vi "Core-Init.vi"(10 "Class Return Notifier":refnum<notifier>, 11 "Engine in":refnum<class "Engine.lvclass">) -> (0 "error out":errorcluster, 3 "Engine out":refnum<class "Engine.lvclass">)   [LabVIEW 2024, in "GLF.lvlib" / "Engine.lvclass"]
uses:
  Engine.lvclass
  IAmGLF/IAmGLF.lvclass
  Window/Window.lvclass
  Engine.lvclass/Engine.ctl
  C:/Users/saukko/Dev/GLF/Sources/GLF/IAmEngine/IAmEngine.lvclass
  C:/Users/saukko/Dev/GLF/Sources/GLF/IAmGLF/IAmGLF.lvclass
  C:/Users/saukko/Dev/GLF/Sources/GLF/Engine/Engine.lvclass
  <vilib>/Saukko/LV SDL3/Sources/SDL3/Init/Init.lvlib
  Command--enum.ctl
  Command--cluster.ctl
  <vilib>/Saukko/LV SDL3/Sources/SDL3/Init/InitFlags--ring.ctl
  <vilib>/Saukko/LV SDL3/Sources/SDL3/Video/Video.lvlib
  DVR--cluster.ctl
  Metrics--cluster.ctl
  Context--cluster.ctl
  Config--cluster.ctl
  VSync--enum.ctl
  Command--queue.ctl
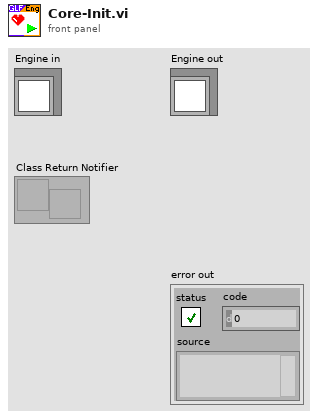
[diagram p1: front panel]
types:
  T1 = typedef "GLF.lvlib/Engine.lvclass/VSync--enum.ctl" = enum16{"Disabled", "Enabled", "Adaptative"}
  T2 = typedef "GLF.lvlib/Engine.lvclass/DVR--cluster.ctl" = cluster{"CMD Queue":T3, "Config":T4, "Ctxt":T5, "Metrics":T6, "GLF Instances":set{refnum<class "IAmGLF.lvclass">}, "Window Instances":map{i64, refnum<class "Window.lvclass">}}
  T3 = typedef "GLF.lvlib/Engine.lvclass/Command--queue.ctl" = refnum<queue>
  T4 = typedef "GLF.lvlib/Engine.lvclass/Config--cluster.ctl" = cluster{"Quit On Last Window Closed":bool, "VSync":T1, "FPS Target":dbl}
  T5 = typedef "GLF.lvlib/Engine.lvclass/Context--cluster.ctl" = cluster{"Ticks Begin":u64, "VSync Enabled":bool}
  T6 = typedef "GLF.lvlib/Engine.lvclass/Metrics--cluster.ctl" = cluster{"Uptime [ms]":u64, "Loop Time [ms]":u64}
  T7 = typedef "SDL3.lvlib/Init.lvlib/InitFlags--ring.ctl" = u32
  T8 = typedef "GLF.lvlib/Engine.lvclass/Command--cluster.ctl" = cluster{"Cmd":T9, "Data":variant}
  T9 = typedef "GLF.lvlib/Engine.lvclass/Command--enum.ctl" = enum16{"Quit", "Register Window"}
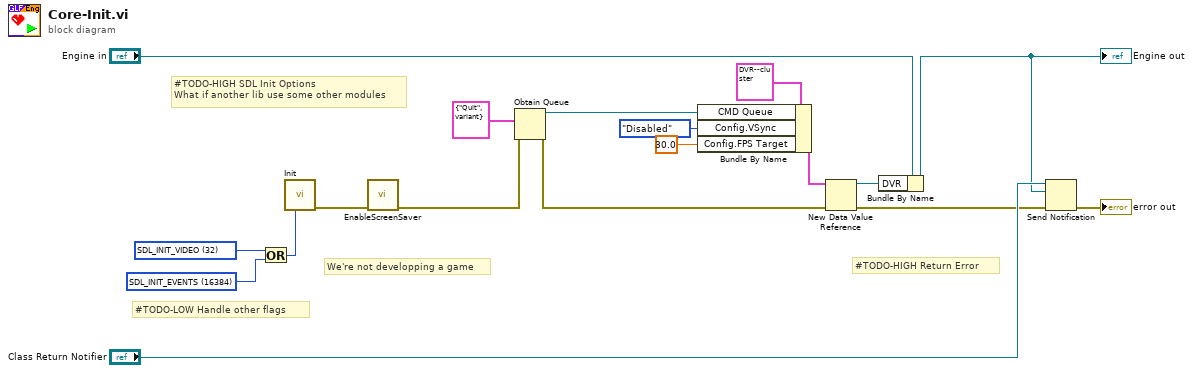
[diagram p0: block diagram]
diagram:
  w14 = T7 16384 items=["NONE"=0, "SDL_INIT_AUDIO"=16, "SDL_INIT_VIDEO"=32, "SDL_INIT_JOYSTICK"=512, "SDL_INIT_HAPTIC"=4096, "SDL_INIT_GAMEPAD"=8192, "SDL_INIT_EVENTS"=16384, "SDL_INIT_SENSOR"=32768, "SDL_INIT_CAMER"=65536] ("y")
  w16 = T7 32 items=["NONE"=0, "SDL_INIT_AUDIO"=16, "SDL_INIT_VIDEO"=32, "SDL_INIT_JOYSTICK"=512, "SDL_INIT_HAPTIC"=4096, "SDL_INIT_GAMEPAD"=8192, "SDL_INIT_EVENTS"=16384, "SDL_INIT_SENSOR"=32768, "SDL_INIT_CAMER"=65536] ("InitFlags")
  # "#TODO-HIGH Return Error"
  # "#TODO-LOW Handle other flags"
  # "We're not developping a game"
  # "#TODO-HIGH SDL Init Options\nWhat if another lib use some other modules"
  n1 = Or(x=w16, y=w14) -> (x .or. y?=w15:T7)
  n2 = call <vilib>:"Init.vi"("InitFlags"=w15) -> ("error out"=w17:errorcluster)  [unwired: 10 in]
  n3 = call <vilib>:"EnableScreenSaver.vi"("No Error"=w17) -> ("Error Out"=w10:errorcluster)  [unwired: 10 in]
  n4 = Obtain Queue(element data type=T8 {"Cmd"=enum."Quit", "Data"=variant} ("Command"), error in (no error)=w10) -> (queue out=w12:refnum<queue>, error out=w6:errorcluster)  [unwired: 3 in, 1 out]
  n5 = Bundle By Name(cluster=T2 {"CMD Queue"=refnum, "Config"={"Quit On Last Window Closed"=FALSE, "VSync"=enum."Disabled", "FPS Target"=0.0}, "Ctxt"={"Ticks Begin"=0, "VSync Enabled"=FALSE}, "Metrics"={"Uptime [ms]"=0, "Loop Time [ms]"=0}, "GLF Instances"={}, "Window Instances"={}} ("DVR"), "CMD Queue"=w12, "Config.VSync"=VSync--enum."Disabled", "Config.FPS Target"=30.0) -> (w5:T2)
  n6 = New Data Value Reference(data value=w5, error in=w6) -> (data value reference=w4:refnum<data-value>, error out=w1:errorcluster)
  n7 = Bundle By Name(cluster="Engine in", "DVR"=w4) -> (w2:refnum<class "Engine.lvclass">)
  "Engine out" <- w2
  n8 = Send Notification(notification=w2, notifier="Class Return Notifier", error in (no error)=w1) -> (error out=→"error out":errorcluster)  [unwired: 1 out]
